vi "2.4.vi"() -> ()   [LabVIEW 2020]
panel:
  out "division":string
  out "multiplicacion":string
  out "resta":string
  out "suma":string
  in  "Y":dbl
  in  "X":dbl
  # "INGRESE SUS DATOS"
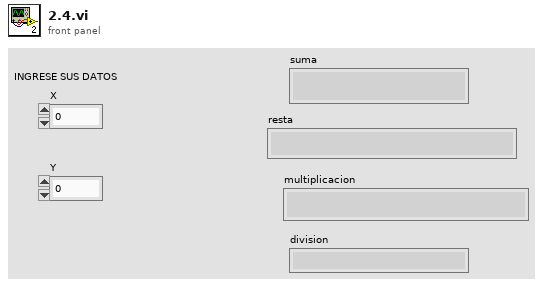
[diagram p1: front panel]
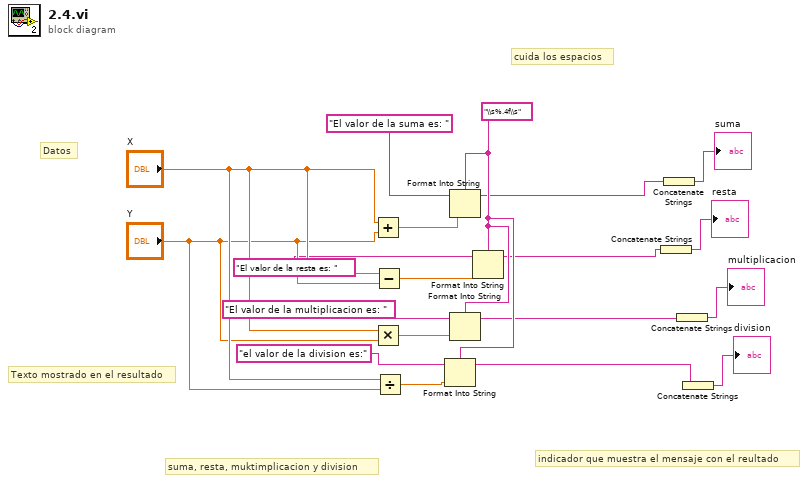
[diagram p0: block diagram]
diagram:
  w9 = "\\s%.4f\\s" ("format string")
  # "indicador que muestra el mensaje con el reultado"
  # "cuida los espacios"
  # "Texto mostrado en el resultado"
  # "suma, resta, muktimplicacion y division"
  # "Datos"
  n1 = Add(x="X", y="Y") -> (x+y=w17:dbl)
  n2 = Multiply(x="X", y="Y") -> (x*y=w12:dbl)
  n3 = Subtract(x="X", y="Y") -> (x-y=w14:dbl)
  n4 = Divide(x="X", y="Y") -> (x/y=w10:dbl)
  n5 = Format Into String(format string=w9, initial string="el valor de la division es:", w10) -> (resulting string=w1:string)  [unwired: 1 in, 1 out]
  n6 = Format Into String "Format Into String"(format string=w9, initial string="El valor de la suma es: ", w17) -> (resulting string=w8:string)  [unwired: 1 in, 1 out]
  n7 = Format Into String(format string=w9, initial string="El valor de la multiplicacion es: ", w12) -> (resulting string=w2:string)  [unwired: 1 in, 1 out]
  n8 = Format Into String(format string=w9, initial string="El valor de la resta es: ", w14) -> (resulting string=w3:string)  [unwired: 1 in, 1 out]
  n9 = Concatenate Strings(w3) -> (→"resta":string)
  n10 = Concatenate Strings "Concatenate Strings"(w8) -> (→"suma":string)
  n11 = Concatenate Strings(w2) -> (→"multiplicacion":string)
  n12 = Concatenate Strings(w1) -> (→"division":string)
